vi "setTriggeredMode.vi"(8 "error in (no error)":errorcluster, 11 "pHandle":u32) -> (0 "error out":errorcluster, 2 "return type":i32)   [LabVIEW 2011, in "sbgLabView.lvlib"]
uses:
  sbgLabView.lvlib
  sbgMatLab.dll
panel:
  in  "outputMaskStr":string
  in  "triggerMaskStr":string
  in  "condId":u8
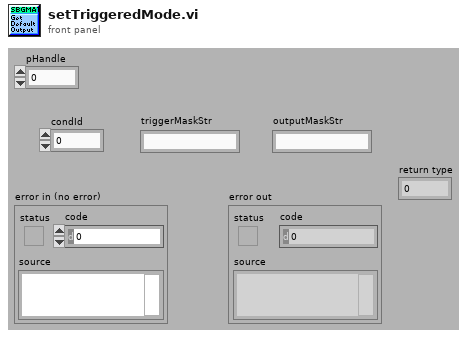
[diagram p1: front panel]
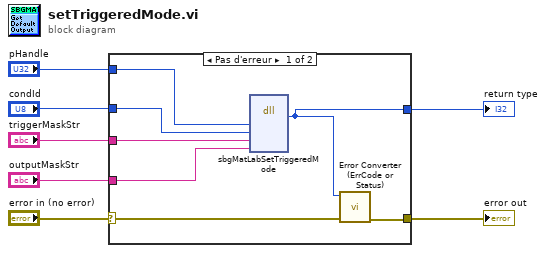
[diagram p0: block diagram]
diagram:
  n1 = case shown="Pas d'erreur" "error in (no error)" {
    selector: "error in (no error)" -> [w12 w15]
    tunnel: [w11 w15] -> w6
    tunnel: [w14 _] -> w5
    tunnel: "pHandle" -> [w13 _]
    tunnel: "condId" -> [w10 _]
    tunnel: "triggerMaskStr" -> [w9 _]
    tunnel: "outputMaskStr" -> [w8 _]
    frame No Error {
      n2 = dll-call lib="C:/SBG-Systems/remote/projects/software/projects/labviewExample/sbgLabView/sbgMatLab.*" fn="sbgMatLabSetTriggeredMode" ("sbgMatLab.dll:sbgMatLabGetDefaultOutputMask")("pHandle"=w13, "condId"=w10, "triggerMaskStr"=w9, "outputMaskStr"=w8) -> ("type de retour"=w14:i32)  [unwired: 7 in, 2 out]
      n3 = call "Error Converter (ErrCode or Status).vi"("error in (no error)"=w12, "error code"=w14) -> ("error out"=w11:errorcluster)  [unwired: 9 in]
    }
    frame Error {
    }
  }
  "return type" <- w5
  "error out" <- w6
